vi "Teleop.vi"(10 "Match Info":T1={"Autonomous Elapsed Seconds"=0.0, "TeleOp Elapsed Seconds"=0.0, "Disabled Elapsed Seconds"=0.0, "Visited Autonomous"=FALSE, "Visited TeleOp"=FALSE, "Visited Disabled"=FALSE, "Autonomous Settings"={"Autonomous Style"=enum."Independent", "VI Refnum"=refnum}}, 11 "Call Context":T2) -> ()   [LabVIEW 2019]
doc: "This VI is called for each TeleOp packet received from the DS where the robot is not disabled. It is often used to read from the joysticks and update I/O or to update setpoints for timed control loops. It should complete and return within 20 milliseconds or it may miss DS packets."
uses:
  <vilib>/Rock Robotics/WPI/DriverStation/WPI_DriverStationDerivedRobotMode.ctl
  <vilib>/Rock Robotics/WPI/DriverStation/WPI_DriverStationMatch Info.ctl
  <vilib>/Rock Robotics/WPI/Utilities/WPI_GetSetVariantRefNum.vi
  <vilib>/Rock Robotics/Network Tables/SD Write Boolean Array.vi
  <vilib>/Rock Robotics/Network Tables/SD Write Numeric Array.vi
  Robot Global Data.vi
  <vilib>/Rock Robotics/Network Tables/NT Write Number.vi
  <vilib>/Rock Robotics/Network Tables/NT Read Number.vi
  <vilib>/Rock Robotics/Network Tables/NT Read Boolean.vi
panel:
  out "Right":cluster{"Left Motor Value":dbl, "output":dbl}(graph)
  out "Left":cluster{"Left Motor Value":dbl, "output":dbl}(graph)
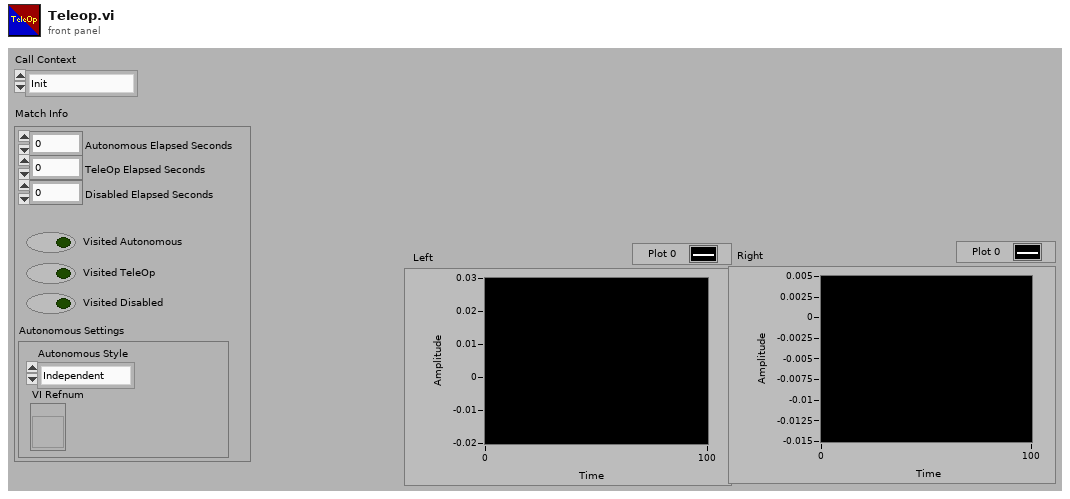
[diagram p1: front panel]
types:
  T1 = typedef "WPI_DriverStationMatch Info.ctl" = cluster{"Autonomous Elapsed Seconds":dbl, "TeleOp Elapsed Seconds":dbl, "Disabled Elapsed Seconds":dbl, "Visited Autonomous":bool, "Visited TeleOp":bool, "Visited Disabled":bool, "Autonomous Settings":cluster{"Autonomous Style":enum16{"Iterative", "Independent"}, "VI Refnum":refnum<vi>}}
  T2 = typedef "WPI_DriverStationDerivedRobotMode.ctl" = enum16{"Init", "Execute", "Stop"}
  T3 = typedef "WPI_JoystickDevRef.ctl" = cluster{"Device":T4}
  T4 = typedef "WPI_JoystickDeviceEnum.ctl" = enum16{"USB 0", "USB 1", "USB 2", "USB 3", "USB 4", "USB 5"}
  T5 = typedef "WPI_RobotDriveDevRef.ctl" = cluster{"DevStatus":errorcluster, "Motors[]":T6[], "Square Inputs":bool, "Max Output":dbl}
  T6 = typedef "WPI_MotorControlDeviceRef.ctl" = cluster{"DeviceStatus":errorcluster, "Type":T7, "PWM":cluster{"PWM Channel":T8, "DeadBand":T9}, "CAN":cluster{"Device Number":u8, "SetOutput VI Ref":variant, "GetOutput VI Ref":variant, "Enable VI Ref":variant, "Disable VI Ref":variant, "Data":variant}, "Invert":bool, "DIO PWM":cluster{"PWM \"Enable\" Channel":T8, "DIOChannel":T10, "PWM Rate":dbl}}
  T7 = typedef "WPI_MotorControlType.ctl" = enum16{"PWM", "CAN", "DIO PWM"}
  T8 = typedef "FPGA_DIOPWMChannel.ctl" = enum8{"PWM 0", "PWM 1", "PWM 2", "PWM 3", "PWM 4", "PWM 5", "PWM 6", "PWM 7", "PWM 8", "PWM 9", "PWM MXP 0", "PWM MXP 1", "PWM MXP 2", "PWM MXP 3", "PWM MXP 4", "PWM MXP 5", "PWM MXP 6", "PWM MXP 7", "PWM MXP 8", "PWM MXP 9", "Invalid"}
  T9 = typedef "WPI_PWMDeadband.ctl" = cluster{"Name":string, "maxPositivePwm":i32, "minPositivePwm":i32, "centerPwm":i32, "maxNegativePwm":i32, "minNegativePwm":i32, "angularRange":u16}
  T10 = typedef "FPGA_DIOChannel.ctl" = enum8{"DIO 0", "DIO 1", "DIO 2", "DIO 3", "DIO 4", "DIO 5", "DIO 6", "DIO 7", "DIO 8", "DIO 9", "DIO MXP 0", "DIO MXP 1", "DIO MXP 2", "DIO MXP 3", "DIO MXP 4", "DIO MXP 5", "DIO MXP 6", "DIO MXP 7", "DIO MXP 8", "DIO MXP 9", "DIO MXP 10", "DIO MXP 11", "DIO MXP 12", "DIO MXP 13", "DIO MXP 14", "DIO MXP 15", "SPI Port CS1", "SPI Port CS2", "SPI Port CS3", "SPI Port MISO", "SPI Port MOSI", "Invalid"}
  T11 = typedef "WPI_ServoDeviceRef.ctl" = cluster{"DeviceStatus":errorcluster, "PWM Channel":T8, "DeadBand":T9}
  T12 = cluster{"Left Motor Value":dbl, "Right Motor Value":dbl}
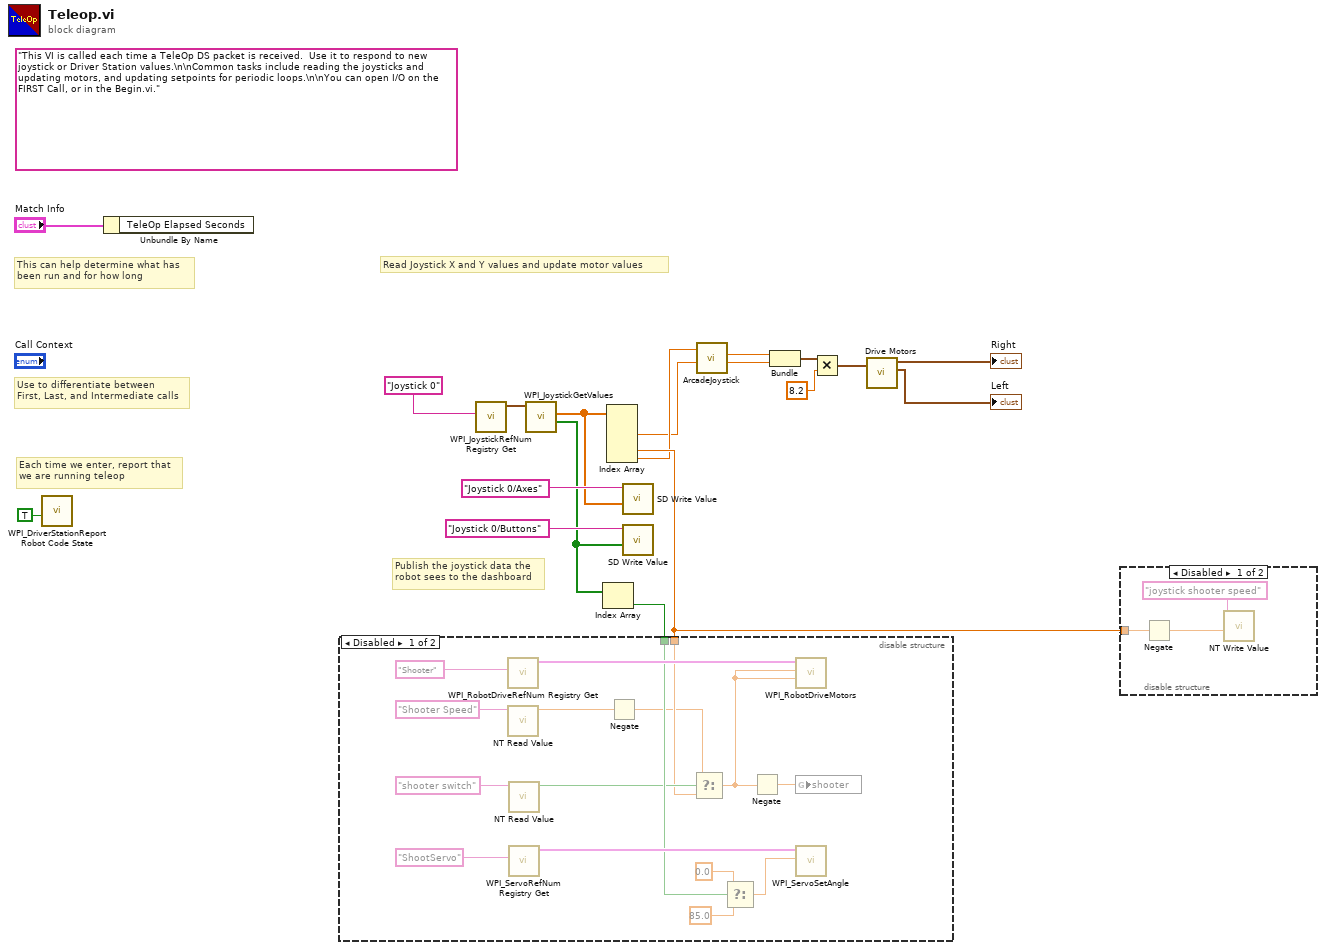
[diagram p0: block diagram]
diagram:
  (unwired) "This VI is called each time a TeleOp DS packet is received.  Use it to respond to new joystick or Driver Station values.\n\nCommon tasks include reading the joysticks and updating motors, and updating setpoints for periodic loops.\n\nYou can open I/O on the FIRST Call, or in the Begin.vi."
  # "Publish the joystick data the\nrobot sees to the dashboard"
  # "Each time we enter, report that\nwe are running teleop"
  # "Use to differentiate between\nFirst, Last, and Intermediate calls"
  # "This can help determine what has\nbeen run and for how long"
  # "Read Joystick X and Y values and update motor values"
  n1 = call <vilib>:"WPI_DriverStationReport Robot Code State.vi"("TeleOp"=TRUE ("Autonomous")) -> ()  [unwired: 10 in, 1 out]
  n2 = Unbundle By Name("Match Info") -> ()  [unwired: 1 out]
  n3 = call <vilib>:"WPI_JoystickRefNum Registry Get.vi"("refnum name"="Joystick 0") -> ("JoystickDevRef"=w17:T3)  [unwired: 1 in, 9 out]
  n4 = call <vilib>:"WPI_JoystickGetValues.vi"("JoystickDevRef"=w17) -> ("Buttons"=w12:bool[], "Axes"=w14:dbl[])  [unwired: 6 in, 3 out]
  n5 = Index Array(array=w12) -> (element=w11:bool)  [unwired: 1 in]
  n6 = Index Array(array=w14) -> (element #2=w8:dbl, element #4=w10:dbl, element #5=w9:dbl)  [unwired: 5 in, 2 out]
  n7 = disable-structure shown="Disabled" {
    disable-tunnel: w11 -> [w30 _]
    disable-tunnel: w10 -> [w22 _]
    frame Disabled {
      n8 = call <vilib>:"WPI_RobotDriveRefNum Registry Get.vi"("refnum name"="Shooter") -> ("RobotDriveDevRef"=w33:T5)  [unwired: 9 in, 1 out]
      n9 = call-poly <vilib>:"NT Read Value.vi"("Name"="Shooter Speed") -> ("Numeric"=w23:dbl)  [unwired: 9 in, 1 out]
      n10 = call-poly <vilib>:"NT Read Value.vi"("Name"="shooter switch" ("refnum name")) -> ("Boolean"=w26:bool)  [unwired: 9 in, 1 out]
      n11 = call <vilib>:"WPI_ServoRefNum Registry Get.vi"("refnum name"="ShootServo") -> ("ServoDeviceRef"=w31:T11)  [unwired: 9 in, 1 out]
      n12 = Negate(x=w23) -> (-x=w21:dbl)
      n13 = Select(t=w21, s=w26, f=w22) -> (s? t:f=w24:dbl)
      n14 = Select(t=0.0 ("y"), s=w30, f=85.0 ("y")) -> (s? t:f=w27:dbl)
      n15 = Negate(x=w24) -> (-x=w20:dbl)
      n16 = call <vilib>:"WPI_RobotDriveMotors.vi"("RightSpeed"=w24, "LeftSpeed"=w24, "RobotDriveDevRef"=w33) -> ()  [unwired: 6 in, 3 out]
      n17 = global write "Robot Global Data.vi" "shooter"(w20) -> ()
      n18 = call <vilib>:"WPI_ServoSetAngle.vi"("Angle"=w27, "ServoDeviceRef"=w31) -> ()  [unwired: 8 in, 2 out]
    }
    frame Enabled {
    }
  }
  n19 = call-poly <vilib>:"SD Write Value.vi"("Numeric Array"=w14, "Name"="Joystick 0/Axes") -> ()  [unwired: 8 in, 2 out]
  n20 = call-poly <vilib>:"SD Write Value.vi"("Boolean Array"=w12, "Name"="Joystick 0/Buttons") -> ()  [unwired: 8 in, 2 out]
  n21 = call "ArcadeJoystick.vi"("Y axis value"=w8, "X axis value"=w9) -> ("Right Motor Value"=w7:dbl, "Left Motor Value"=w4:dbl)  [unwired: 8 in]
  n22 = Bundle("Left Motor Value"=w4, "Right Motor Value"=w7) -> (w6:T12)  [unwired: 1 in]
  n23 = Multiply(x=w6, y=8.2) -> (x*y=w1:T12)
  n24 = call "Drive Motors.vi"("Cluster"=w1) -> ("Left"=→"Left":cluster{"Left Motor Value":dbl, "output":dbl}, "Right"=→"Right":cluster{"Left Motor Value":dbl, "output":dbl})  [unwired: 9 in]
  n25 = disable-structure shown="Disabled" {
    disable-tunnel: w10 -> [w37 _]
    frame Disabled {
      n26 = Negate(x=w37) -> (-x=w36:dbl)
      n27 = call-poly <vilib>:"NT Write Value.vi"("Numeric"=w36, "Name"="joystick shooter speed") -> ()  [unwired: 9 in, 1 out]
    }
    frame Enabled {
    }
  }
